vi "Pre Launch Init.vi"(11 "Cooler UI with Events in":refnum<class "Cooler UI with Events.lvclass">) -> (0 "error out":errorcluster, 3 "Cooler UI with Events out":refnum<class "Cooler UI with Events.lvclass">)   [LabVIEW 2012, in "Cooler UI.lvlib" / "Cooler UI with Events.lvclass"]
doc: "Defines behavior that occurs after the Launch Actor.vi method is invoked but before the actor actually launches. This method is guaranteed to finish before Launch Actor.vi returns to its caller. Any resources this VI obtains are guaranteed to have the same lifetime as the actor itself.\n\nBy default, this method does nothing. A descendant class may override it to define behavior."
uses:
  Cooler UI with Events.lvclass
  Status.ctl
  Cooler UI with Events.lvclass/Cooler UI with Events.ctl
  <vilib>/ActorFramework/Actor/Actor.lvclass
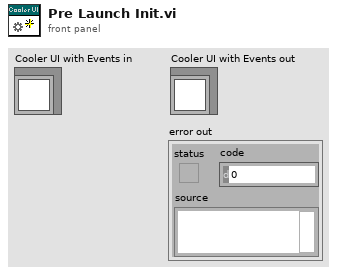
[diagram p1: front panel]
types:
  T1 = typedef "Cooler UI.lvlib/Cooler UI with Events.lvclass/Status.ctl" = cluster{"Fan A":cluster{"State":bool, "Fault":bool}, "Fan B":cluster{"State":bool, "Fault":bool}}
  T2 = cluster{"Fan Status":refnum<user-event>, "Temperature":refnum<user-event>, "Pump":refnum<user-event>}
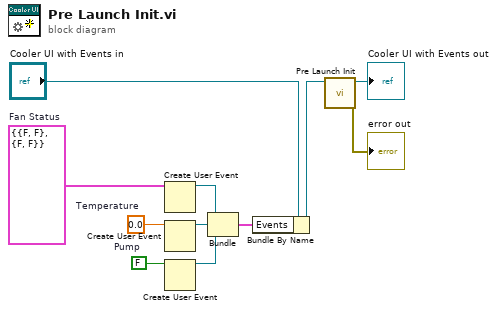
[diagram p0: block diagram]
diagram:
  w4 = T1 {"Fan A"={"State"=FALSE, "Fault"=FALSE}, "Fan B"={"State"=FALSE, "Fault"=FALSE}}  # Fan Status
  w7 = FALSE  # Pump
  w6 = 0.0  # Temperature
  n1 = Create User Event(user event datatype=w4) -> (user event=w8:refnum<user-event>)  [unwired: 1 in, 1 out]
  n2 = Create User Event(user event datatype=w6) -> (user event=w9:refnum<user-event>)  [unwired: 1 in, 1 out]
  n3 = Create User Event(user event datatype=w7) -> (user event=w10:refnum<user-event>)  [unwired: 1 in, 1 out]
  n4 = Bundle("Fan Status"=w8, "Temperature"=w9, "Pump"=w10) -> (w5:T2)  [unwired: 1 in]
  n5 = Bundle By Name(cluster="Cooler UI with Events in", "Events"=w5) -> (w2:refnum<class "Cooler UI with Events.lvclass">)
  n6 = call-parent "Pre Launch Init.vi"("Actor in"=w2) -> ("error out"=→"error out":errorcluster, "Actor out"=→"Cooler UI with Events out":refnum<class "Cooler UI with Events.lvclass">)  [unwired: 9 in]
